vi "Get Dependency.vi"(8 "error in (no error)":errorcluster, 11 "Application in":refnum<class "Application.lvclass">) -> (0 "error out":errorcluster, 2 "Dependency":T1, 3 "Application out":refnum<class "Application.lvclass">)   [LabVIEW 2019, in "Application.lvclass"]
doc: "Developed by Kevin Thompson\nkevin@thompsonengineering.net\n\nCopyright 2018\nThompson Engineering, LLC"
uses:
  Application.lvclass
  DataTypes/Dependency--cluster.ctl
  Subsystems/Main/Main.lvclass
  Subsystems/Config/Config.lvclass
  Common/ErrorHandler/ErrorHandler.lvclass
  Subsystems/DAQ_Engine/DAQ_Engine.lvclass
  Subsystems/Log_Engine/Log_Engine.lvclass
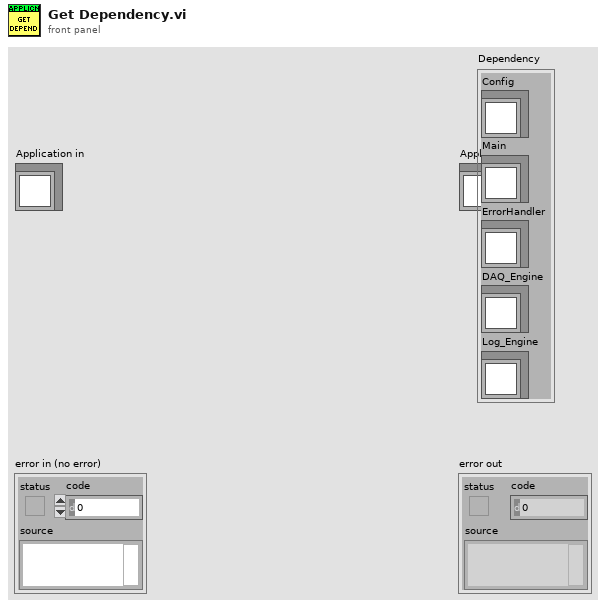
[diagram p1: front panel]
types:
  T1 = typedef "Application.lvclass/Dependency--cluster.ctl" = cluster{"Config":refnum<class "Config.lvclass">, "Main":refnum<class "Main.lvclass">, "ErrorHandler":refnum<class "ErrorHandler.lvclass">, "DAQ_Engine":refnum<class "DAQ_Engine.lvclass">, "Log_Engine":refnum<class "Log_Engine.lvclass">}
  T2 = typedef "Application.lvclass/ObjData--cluster.ctl" = cluster{"Settings":T3, "Public Events":T4, "Dependency":T1, "ReadData-placeholder":T5, "VISA-placeholder":refnum<visa-resource-name>, "Subsys ClassRefs Dict":T6, "InverterWaveformsQ":T7, "RawDaqDataQ":T8}
  T3 = typedef "Application.lvclass/Settings--cluster.ctl" = cluster{"Simulation":bool}
  T4 = typedef "Application.lvclass/Public Events--cluster.ctl" = cluster{"Application.AsyncCmd Event":refnum<user-event>, "Application.AsyncMsg Event":refnum<user-event>, "stop process":refnum<user-event>}
  T5 = typedef "Application.lvclass/Read Data--cluster.ctl" = cluster{"Data":dbl}
  T6 = typedef "TD Dynamic CVT DVR--ref.ctl" = refnum<data-value>
  T7 = typedef "InverterWaveforms--QRef.ctl" = refnum<queue>
  T8 = typedef "RawDAQDataQRef--cluster.ctl" = refnum<queue>
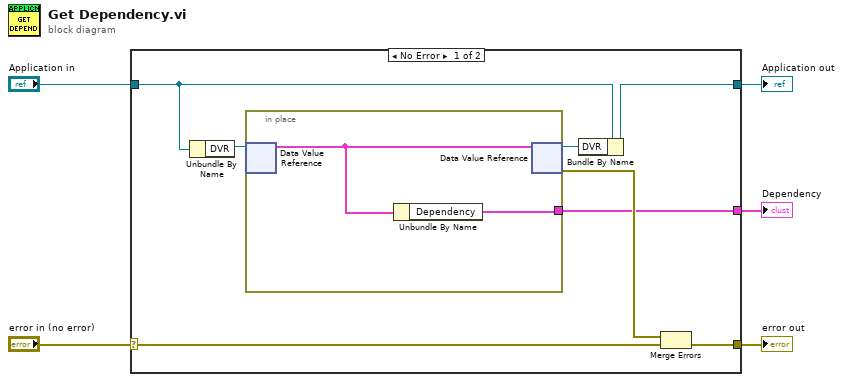
[diagram p0: block diagram]
diagram:
  n1 = case shown="No Error" "error in (no error)" {
    selector: "error in (no error)" -> [w10 w16]
    tunnel: [w6 w16] -> w4
    tunnel: [w9 w17] -> w2
    tunnel: "Application in" -> [w8 w17]
    tunnel: [w7 _] -> w1
    frame No Error {
      n2 = Unbundle By Name(w8) -> ("DVR"=w12:refnum<data-value>)
      n3 = in-place {
        in-place-border: [w14] -> w7
        n4 = in-place-dvr #1(w12) -> (w15:T2)  [unwired: 1 out]
        n5 = Unbundle By Name(w15) -> ("Dependency"=w14:T1)
        n6 = in-place-dvr #1(w15) -> (w13:refnum<data-value>, w11:errorcluster)
      }
      n7 = Bundle By Name(cluster=w8, "DVR"=w13) -> (w9:refnum<class "Application.lvclass">)
      n8 = Merge Errors(w11, w10) -> (w6:errorcluster)
    }
    frame Error {
    }
  }
  "error out" <- w4
  "Application out" <- w2
  "Dependency" <- w1
